vi "AlazarSetLED.vi"(3 "error in (no error)":errorcluster, 4 "State":bool, 5 "Handle":u64) -> (0 "error out":errorcluster, 1 "Return Code":u32, 2 "Handle":u64)   [LabVIEW 2009]
doc: "Control LED on a board's PCI/PCIe mounting bracket."
uses:
  ATSApi.dll
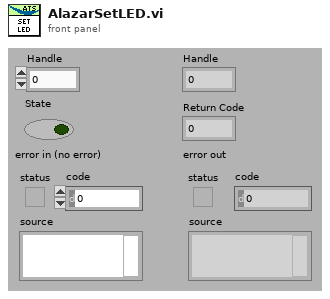
[diagram p1: front panel]
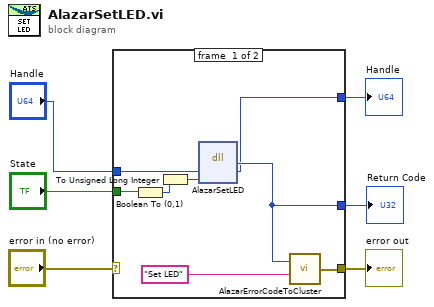
[diagram p0: block diagram]
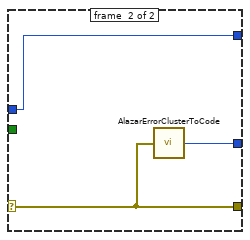
[diagram p2: hidden frame]
diagram:
  n1 = case shown="No Error" "error in (no error)" {
    selector: "error in (no error)" -> [_ w17]
    tunnel: [w11 w17] -> w5
    tunnel: [w13 w16] -> w4
    tunnel: "Handle" -> [w14 w15]
    tunnel: [w10 w15] -> w2
    tunnel: "State" -> [w9 _]
    frame #0 {
      n2 = Boolean To (0,1)(Boolean=w9) -> (0, 1=w8:i16)
      n3 = To Unsigned Long Integer(number=w8) -> (unsigned 32bit integer=w7:u32)
      n4 = dll-call lib="ATSApi.dll" fn="AlazarSetLED"("handle"=w14, "ledON"=w7) -> ("return type"=w13:u32, "handle"=w10:u64)  [unwired: 4 in, 2 out]
      n5 = call "AlazarErrorCodeToCluster.vi"("Message"="Set LED", "Error Code"=w13) -> ("error out"=w11:errorcluster)
    }
    frame #1 {
      n6 = call "AlazarErrorClusterToCode.vi"("error in (no error)"=w17) -> ("Error Code"=w16:u32)
    }
  }
  "Handle" <- w2
  "error out" <- w5
  "Return Code" <- w4
